vi "ARCH_EDITOR_prepare_INSERT_statement.vi"(8 "error_in":errorcluster, 10 "selected_record":i32, 11 "ARCH_EDIT_records":string[][](array[string])) -> (0 "error_out":errorcluster, 3 "INSERT_statement":string)   [LabVIEW 2019]
uses:
  FGV/ARCH_EDITOR_records_display/FGV_ARCH_EDITOR_records_display.ctl
  <userlib>/_OpenG.lib/array/array.llb/Filter 1D Array (String)__ogtk.vi
  <userlib>/_OpenG.lib/array/array.llb/Delete Elements from 1D Array (String)__ogtk.vi
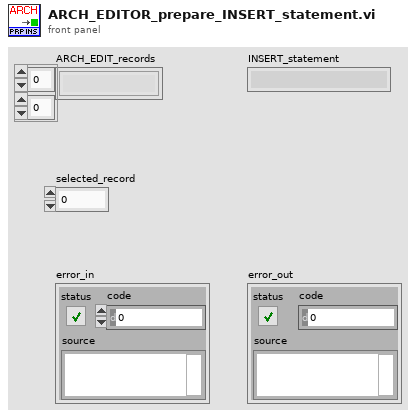
[diagram p1: front panel]
types:
  T1 = typedef "FGV_ARCH_EDITOR_records_display.ctl" = enum16{"initialize", "set_arch_cfg_tables_names", "set_station_number", "set_type_filter", "set_headers", "set_records", "get_arch_cfg_table_name", "get_arch_cfg_hist_table_name", "get_station_number", "get_type_filter", "get_headers", "get_uneditable_columns", "get_all_info", "record_added?", "record_inserted?", "record_edited?", "record_updated?", "record_deleted?", "discard_changes"}
  T2 = typedef "ARCH_EDITOR_all_info.ctl" = cluster{"station_number":string, "type_filter":string, "archivisation_cfg_table":string, "archivisation_cfg_history":string, "column_names":string[], "uneditable_columns":string[], "uneditable_columns":i32[], "editable_columns":i32[], "values_in_database":string[][], "size":cluster{"columns":i32, "SQL_rows":i32, "disp_rows":i32}, "ARCH_record_states":T3[]}
  T3 = typedef "SQL_record_states.ctl" = enum16{"Equal", "Added", "Edited", "Deleted"}
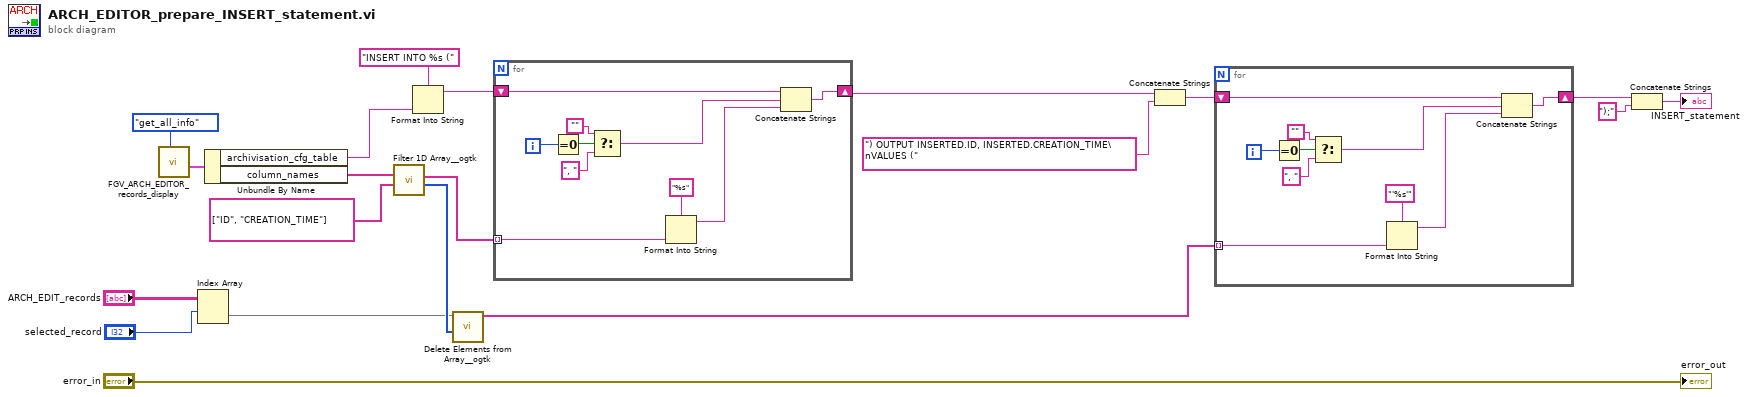
[diagram p0: block diagram]
diagram:
  n1 = call "FGV_ARCH_EDITOR_records_display.vi"("options"=FGV_ARCH_EDITOR_records_display."get_all_info") -> ("all_info"=w8:T2)  [unwired: 7 in, 3 out]
  n2 = Index Array(array="ARCH_EDIT_records", index (row)="selected_record") -> (element=w3:string[])  [unwired: 1 in]
  n3 = Unbundle By Name(w8) -> ("archivisation_cfg_table"=w6:string, "column_names"=w7:string[])
  n4 = call-poly <userlib>:"Filter 1D Array__ogtk.vi"("items to filter"=string[] ["ID", "CREATION_TIME"], "array"=w7) -> ("filtered item indices"=w13:i32[], "filtered array"=w15:string[])  [unwired: 4 in]
  n5 = Format Into String(format string="INSERT INTO %s (", w6) -> (resulting string=w18:string)  [unwired: 2 in, 1 out]
  n6 = call-poly <userlib>:"Delete Elements from Array__ogtk.vi"("indices"=w13, "array"=w3) -> ("array w/ subset deleted"=w12:string[])  [unwired: 8 in, 1 out]
  n7 = for {
    tunnel: w15 -> [w23] mode=indexing
    shift-right: [w25] -> w20
    shift-left: w18 -> [w26]
    i -> [w30]
    n8 = Equal To 0?(x=w30) -> (x = 0?=w29:bool)
    n9 = Select(t="", s=w29, f=", ") -> (s? t:f=w24:string)
    n10 = Format Into String(format string="%s", w23) -> (resulting string=w22:string)  [unwired: 2 in, 1 out]
    n11 = Concatenate Strings(w26, w24, w22) -> (w25:string)
  }
  n12 = Concatenate Strings(w20, ") OUTPUT INSERTED.ID, INSERTED.CREATION_TIME\nVALUES (" ("string")) -> (w14:string)
  n13 = for {
    tunnel: w12 -> [w33] mode=indexing
    shift-right: [w35] -> w10
    shift-left: w14 -> [w36]
    i -> [w40]
    n14 = Equal To 0?(x=w40) -> (x = 0?=w39:bool)
    n15 = Select(t="", s=w39, f=", ") -> (s? t:f=w34:string)
    n16 = Format Into String(format string="'%s'", w33) -> (resulting string=w32:string)  [unwired: 2 in, 1 out]
    n17 = Concatenate Strings(w36, w34, w32) -> (w35:string)
  }
  n18 = Concatenate Strings(w10, ");" ("string")) -> (→"INSERT_statement":string)
  "error_out" <- "error_in"
